vi "GCMPlugin_GetPluginName.vi"(8 "error in (no error)":errorcluster, 11 "TemplatePlugin in":refnum<class "InstallerSpecEditor.lvclass">) -> (0 "error out":errorcluster, 2 "PluginName":string, 3 "TemplatePlugin out":refnum<class "InstallerSpecEditor.lvclass">)   [LabVIEW 2014, in "BuildSpecEditor.lvlib" / "InstallerSpecEditor.lvclass"]
uses:
  InstallerSpecEditor.lvclass
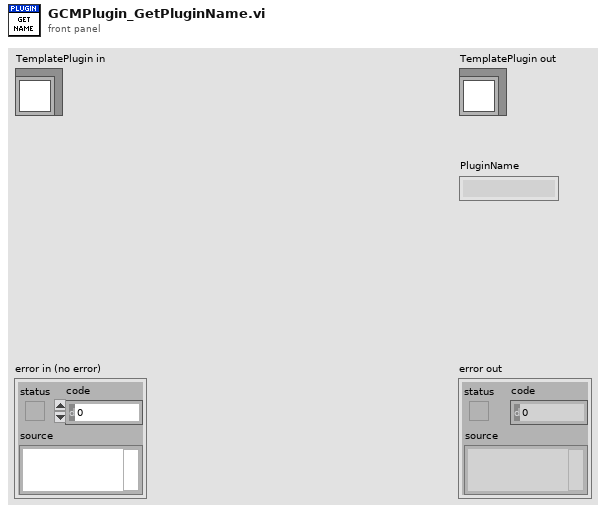
[diagram p1: front panel]
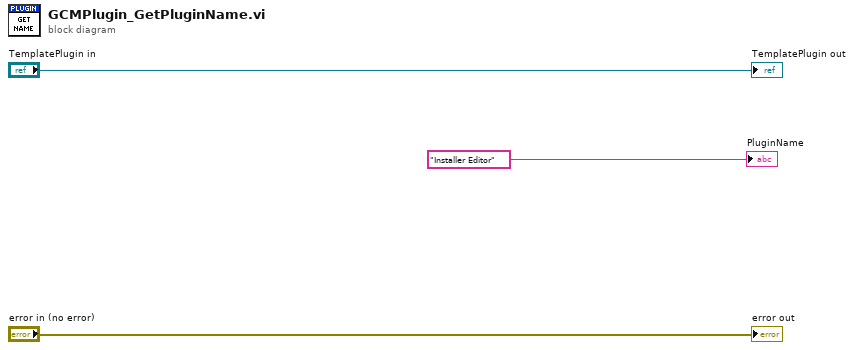
[diagram p0: block diagram]
diagram:
  "error out" <- "error in (no error)"
  "TemplatePlugin out" <- "TemplatePlugin in"
  "PluginName" <- "Installer Editor"
